vi "Find Parent Interface.vi"(8 "error in (no error)":errorcluster, 11 "Mock Class Path":path) -> (0 "error out":errorcluster, 3 "Parent Interface":path)   [LabVIEW 2020, in "Mock Class Updater.lvclass"]
uses:
  Mock Class Updater.lvclass
  Mock Class Updater.lvclass/Mock Class Updater.ctl
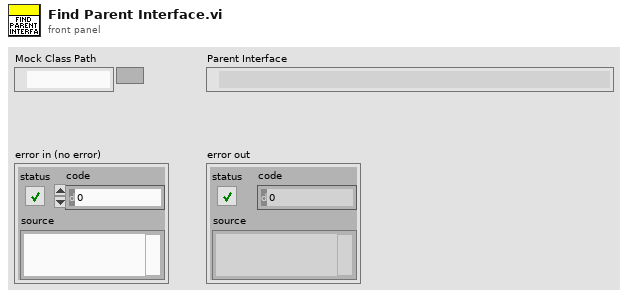
[diagram p1: front panel]
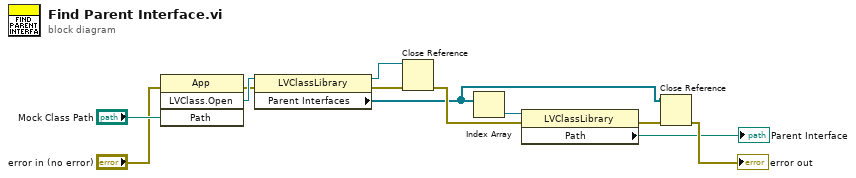
[diagram p0: block diagram]
diagram:
  n1 = invoke class="App" method="LVClass.Open"(error in="error in (no error)", "Path"="Mock Class Path") -> (error out=w4:errorcluster, "LVClass.Open"=w5:refnum<vi>)  [unwired: 2 in, 2 out]
  n2 = property class="LVClassLibrary"(reference=w5, error in=w4) -> (reference out=w11:refnum<vi>, error out=w9:errorcluster, "Parent Interfaces"=w8:refnum<vi>[])
  n3 = Close Reference(reference=w11, error in (no error)=w9) -> (error out=w10:errorcluster)
  n4 = Index Array(array=w8) -> (element=w6:refnum<vi>)  [unwired: 1 in]
  n5 = property class="LVClassLibrary"(reference=w6, error in=w10) -> (error out=w7:errorcluster, "Path"=→"Parent Interface":path)  [unwired: 1 out]
  n6 = Close Reference(reference=w8, error in (no error)=w7) -> (error out=→"error out":errorcluster)
